vi "DE_Preprocess.vi"(4 "stopping state in":T1={"max iterations"=50, "max function calls"=-1, "max time (sec)"=-1.0, "cur function calls"=0, "init tick count"=0}, 5 "function data":variant, 6 "DE settings":T4={"population size"=10, "scale factor"=0.9, "crossover probability"=0.95, "bound mapping method"=1, "mutation method"=0, "crossover method"=0} {"crossover method" items=["Uniform", "Exponential"]; "mutation method" items=["Random", "Either Or", "Best", "Target to Best"]; "bound mapping method" items=["None", "Random between Bounds and Values", "Re-Initialize"]}, 7 "objective and constraint function":refnum<vi>, 8 "error in (no error)":errorcluster, 9 "State In":T2, 10 "Bounds":cluster{"Min":dbl[], "Max":dbl[]}, 11 "Init Parameters":dbl[][](array[numeric])) -> (0 "error out":errorcluster, 1 "State Out":T2, 2 "stopping state out":T1={"max iterations"=50, "max function calls"=-1, "max time (sec)"=-1.0, "cur function calls"=0, "init tick count"=0})   [LabVIEW 2017, in "NI_AAL_GlobalOptimization.lvlib"]
uses:
  <vilib>/gmath/NI_AAL_GlobalOptimization.lvlib
  <vilib>/gmath/GlobalOptimization.llb/DE_Settings.ctl
  <vilib>/gmath/GlobalOptimization.llb/DE_Bound Mapping Method.ctl
  <vilib>/gmath/GlobalOptimization.llb/DE_Mutation Method.ctl
  <vilib>/gmath/GlobalOptimization.llb/DE_Crossover Method.ctl
  <vilib>/gmath/GlobalOptimization.llb/DE_State.ctl
  <vilib>/gmath/GlobalOptimization.llb/DE_Population.ctl
  <vilib>/gmath/GlobalOptimization.llb/DE_Stopping State.ctl
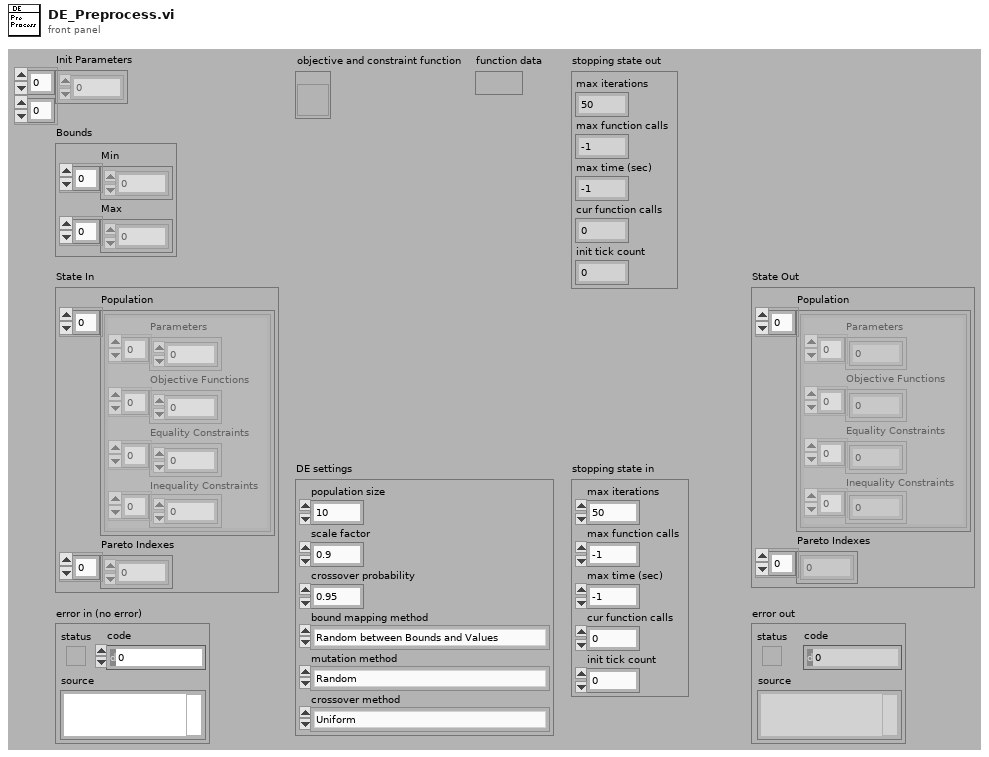
[diagram p1: front panel]
types:
  T1 = typedef "NI_AAL_GlobalOptimization.lvlib/DE_Stopping State.ctl" = cluster{"max iterations":i32, "max function calls":i32, "max time (sec)":dbl, "cur function calls":i32, "init tick count":u32}
  T2 = typedef "NI_AAL_GlobalOptimization.lvlib/DE_State.ctl" = cluster{"Population":T3[], "Pareto Indexes":i32[]}
  T3 = typedef "NI_AAL_GlobalOptimization.lvlib/DE_Population.ctl" = cluster{"Parameters":dbl[], "Objective Functions":dbl[], "Equality Constraints":dbl[], "Inequality Constraints":dbl[]}
  T4 = typedef "NI_AAL_GlobalOptimization.lvlib/DE_Settings.ctl" = cluster{"population size":i32, "scale factor":dbl, "crossover probability":dbl, "bound mapping method":T5, "mutation method":T6, "crossover method":T7}
  T5 = typedef "NI_AAL_GlobalOptimization.lvlib/DE_Bound Mapping Method.ctl" = u16
  T6 = typedef "NI_AAL_GlobalOptimization.lvlib/DE_Mutation Method.ctl" = u16
  T7 = typedef "NI_AAL_GlobalOptimization.lvlib/DE_Crossover Method.ctl" = u16
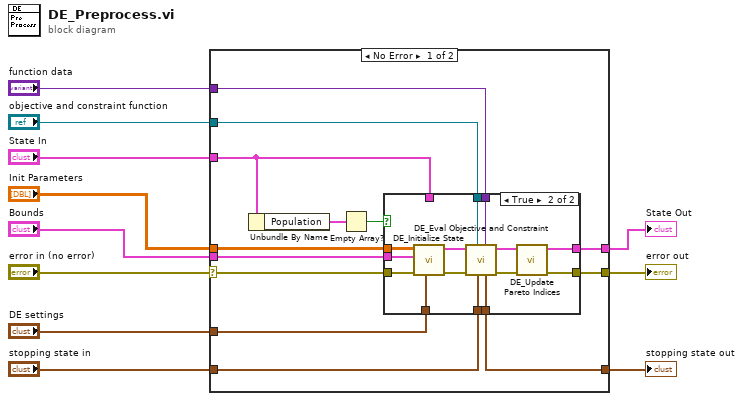
[diagram p0: block diagram]
diagram:
  n1 = case shown="No Error" "error in (no error)" {
    selector: "error in (no error)" -> [w12 w43]
    tunnel: "objective and constraint function" -> [w19 _]
    tunnel: "function data" -> [w24 _]
    tunnel: "DE settings" -> [w22 _]
    tunnel: "Bounds" -> [w23 _]
    tunnel: [w20 _] -> w6
    tunnel: [w18 w43] -> w5
    tunnel: "State In" -> [w15 _]
    tunnel: [w21 w42] -> w3
    tunnel: "Init Parameters" -> [w14 _]
    tunnel: "stopping state in" -> [w13 w42]
    frame No Error {
      n2 = Unbundle By Name(w15) -> ("Population"=w17:T3[])
      n3 = Empty Array?(array=w17) -> (empty?=w16:bool)
      n4 = case shown="True" w16 {
        tunnel: w24 -> [_ w37]
        tunnel: w23 -> [_ w36]
        tunnel: w22 -> [_ w35]
        tunnel: [w26 w29] -> w21
        tunnel: [w27 w34] -> w20
        tunnel: w19 -> [_ w33]
        tunnel: [w25 w32] -> w18
        tunnel: w15 -> [w27 _]
        tunnel: w14 -> [_ w31]
        tunnel: w13 -> [w26 w30]
        tunnel: w12 -> [w25 w28]
        frame False {
        }
        frame True {
          n5 = call <vilib>:"DE_Initialize State.vi"("DE settings"=w35, "error in (no error)"=w28, "Bounds"=w36, "Init Parameters"=w31) -> ("error out"=w39:errorcluster, "State"=w40:T2)  [unwired: 6 in]
          n6 = call <vilib>:"DE_Eval Objective and Constraint.vi"("function data"=w37, "stopping state in"=w30, "objective and constraint function"=w33, "error in (no error)"=w39, "State In"=w40) -> ("error out"=w38:errorcluster, "State Out"=w41:T2, "stopping state out"=w29:T1)  [unwired: 4 in]
          n7 = call <vilib>:"DE_Update Pareto Indices.vi"("error in (no error)"=w38, "State In"=w41) -> ("error out"=w32:errorcluster, "State Out"=w34:T2)  [unwired: 7 in, 1 out]
        }
      }
    }
    frame Error {
    }
  }
  "error out" <- w5
  "State Out" <- w6
  "stopping state out" <- w3
